vi "Read Address Pointer.vi"(8 "INC?":bool, 9 "Load?":bool, 10 "Load Value":u16, 11 "rollover":u16) -> (3 "count":u16)   [LabVIEW 2014]
panel:
  # "Copyright 2014 Vidrio Technologies\nScanImage 5 software is licensed under the Apache License, Version 2.0 (the \"License\"); you may not use any files contained\nwithin the ScanImage 5 release except in compliance with the License. You may obtain a copy of the License at\n http://www.apache.org/licenses/LICENSE-2.0\nUnless required by applicable law or agreed to in writing, software distributed under the License is distributed on an\n\"AS IS\" BASIS, WITHOUT WARRANTIES OR CONDITIONS OF ANY KIND, either express or implied. See the License for the\n specific language governing permissions and limitations under the License."
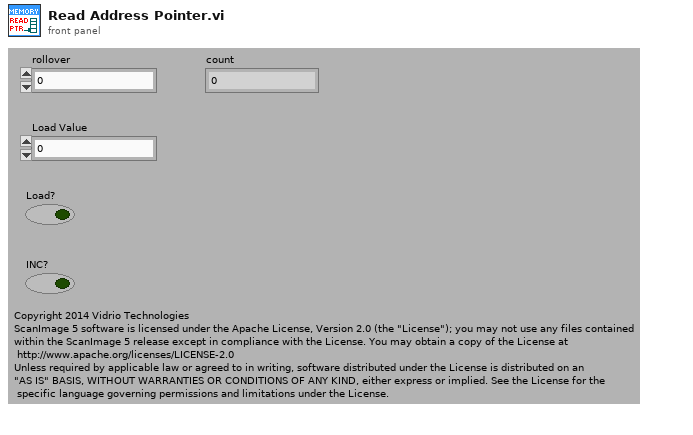
[diagram p1: front panel]
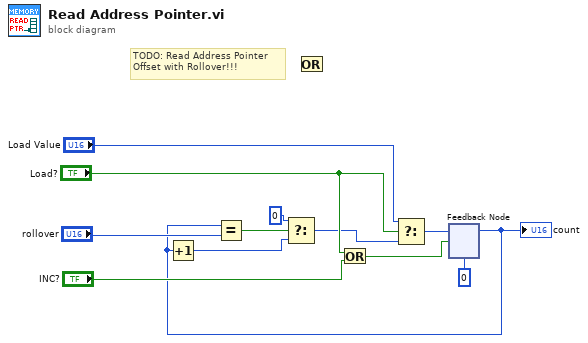
[diagram p0: block diagram]
diagram:
  # "TODO: Read Address Pointer\nOffset with Rollover!!!"
  n1 = Or() -> ()  [unwired: 2 in, 1 out]
  n2 = Or(x="Load?", y="INC?") -> (x .or. y?=w2:bool)
  n3 = feedback #1(u16 0) -> (w1:u16)
  "count" <- w1
  n4 = Increment(x=w1) -> (x+1=w10:u16)
  n5 = Equal?(x=w1, y="rollover") -> (x = y?=w8:bool)
  n6 = Select(t=u16 0, s=w8, f=w10) -> (s? t:f=w4:u16)
  n7 = Select(t="Load Value", s="Load?", f=w4) -> (s? t:f=w3:u16)
  n8 = feedback-in #1(w3, w2) -> ()
